vi "LINC Write Command (Raw).vi"(4 "raw byte offset (default)":i32=-1, 6 "timeout (2000)":u32=2000, 7 "parse only (F)":bool, 8 "error in (no error)":errorcluster, 9 "raw data":string, 10 "packet name":string, 11 "LINC session":refnum<class "LINC.lvclass">) -> (0 "error out":errorcluster, 1 "remote error":bool, 2 "binary command":string, 3 "dup LINC session":refnum<class "LINC.lvclass">)   [LabVIEW 2018, in "STEPkgDriver_LINC.lvlib" / "LINC.lvclass"]
uses:
  LINC.lvclass
  STEPkgDriver_LINC.lvlib
  LINC Global Session Mode.ctl
  LINC Global Config Mode.ctl
  LINC Global Handshake Mode.ctl
  LINC Handshake Internal.ctl
  LINC Global Mode.ctl
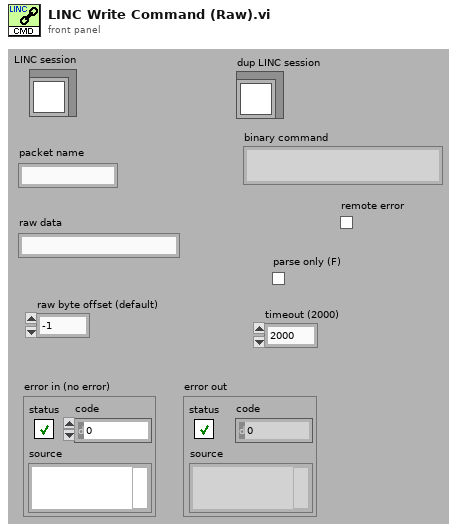
[diagram p1: front panel]
types:
  T1 = typedef "STEPkgDriver_LINC.lvlib/LINC Global Mode.ctl" = enum16{"INIT", "CLEAR", "ADD_PKT_HDR", "ADD_PKT", "GET_PKT_NAMES", "GET_PKT_DESC", "GET_PKT_HDR", "GET_PKT", "SET_PKT", "SET_DATA", "SIM_EN", "SIM_DS"}
  T2 = typedef "STEPkgDriver_LINC.lvlib/LINC Global Config Mode.ctl" = enum16{"INIT", "CLEAR", "SET_CMD_CB", "SET_TLM_CB", "SET_CMD_FIELDS", "SET_TLM_FIELDS", "SET_ID", "GET_CONFIG"}
  T3 = typedef "STEPkgDriver_LINC.lvlib/LINC Handshake Internal.ctl" = cluster{"error":errorcluster, "command data":string}
  T4 = typedef "STEPkgDriver_LINC.lvlib/LINC Global Handshake Mode.ctl" = enum16{"INIT", "CLEAR", "ADD_COMMAND", "RMV_COMMAND", "CLR_HANDSHAKE", "SET_HANDSHAKE", "GET_HANDSHAKE"}
  T5 = typedef "STEPkgDriver_LINC.lvlib/LINC Global Session Mode.ctl" = enum16{"INIT", "CLEAR", "ADD_SESSION", "SET_CONNECTION", "SET_LISTENER", "SET_REFERENCE", "GET_SESSION"}
  T6 = typedef "STEPkgDriver_LINC.lvlib/LINC Config.ctl" = cluster{"cmd callback":refnum<vi>, "tlm callback":refnum<vi>, "cmd ID bitoffset":i32, "cmd ID bitsize":i32, "cmd IDs":i32[], "tlm ID bitoffset":i32, "tlm ID bitsize":i32, "tlm IDs":i32[], "cmd header fields":i32, "tlm header fields":i32, "tlm header size":i32}
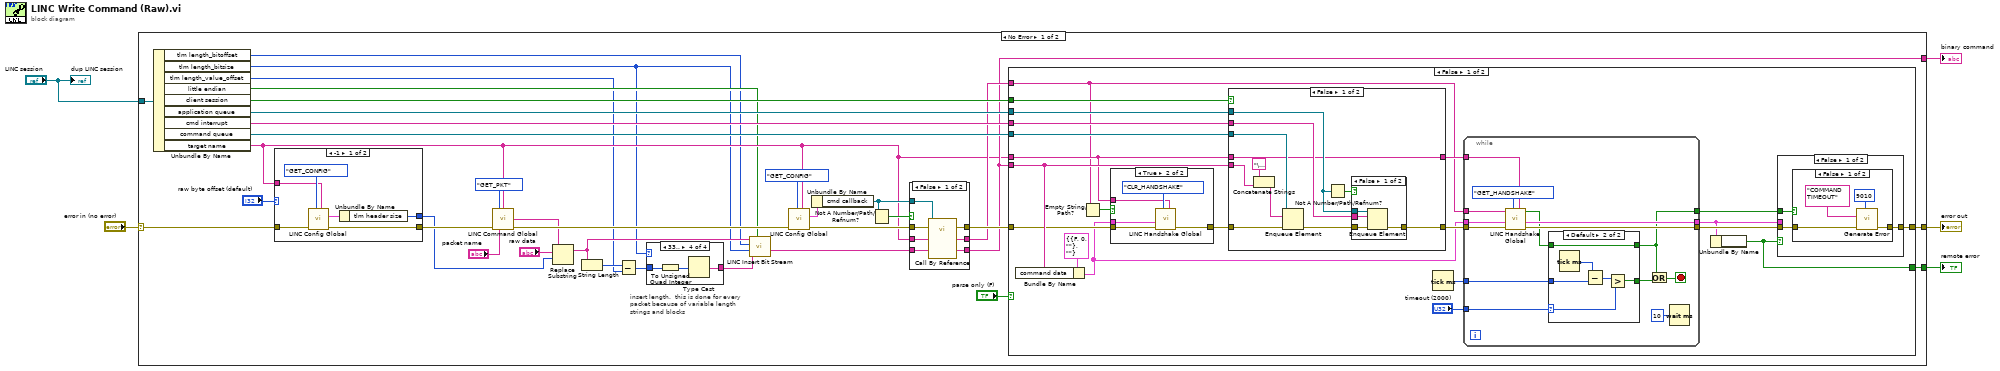
[diagram p0: block diagram]
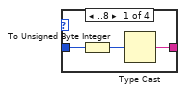
[diagram p2: hidden frame]
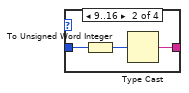
[diagram p3: hidden frame]
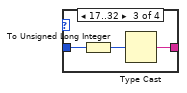
[diagram p4: hidden frame]
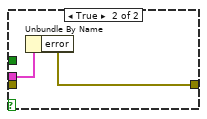
[diagram p8: hidden frame]
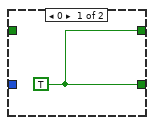
[diagram p10: hidden frame]
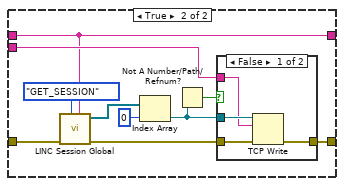
[diagram p12: hidden frame]
diagram:
  n1 = case shown="No Error" "error in (no error)" {
    selector: "error in (no error)" -> [w6 w160]
    tunnel: [w40 w160] -> w5
    tunnel: "LINC session" -> [w38 _]
    tunnel: [w26 _] -> w3
    tunnel: [w7 _] -> w2
    frame No Error {
      # "insert length.  this is done for every packet because of variable length strings and blocks"
      n2 = Unbundle By Name(w38) -> ("tlm length_bitoffset"=w8:i32, "tlm length_bitsize"=w9:i32, "tlm length_value_offset"=w10:i32, "little endian"=w11:bool, "client session"=w37:bool, "application queue"=w36:refnum<queue>, "cmd interrupt"=w35:string, "command queue"=w34:refnum<queue>, "target name"=w17:string)
      n3 = case shown="-1" "raw byte offset (default)" {
        selector: "raw byte offset (default)" -> [_ w59]
        tunnel: [w56 w60] -> w22
        tunnel: w6 -> [w55 w60]
        tunnel: [w54 w59] -> w18
        tunnel: w17 -> [w53 _]
        frame -1 {
          n4 = call "LINC Config Global.vi"("target name"=w53, "mode"=LINC_Global_Config_Mode."GET_CONFIG", "error in (no error)"=w55) -> ("error out"=w56:errorcluster, "config out"=w58:T6)  [unwired: 7 in]
          n5 = Unbundle By Name(w58) -> ("tlm header size"=w54:i32)
        }
        frame Default {
        }
      }
      n6 = call "LINC Command Global.vi"("mode"=LINC_Global_Mode."GET_PKT", "target name"=w17, "error in (no error)"=w22, "packet name"="packet name") -> ("data out"=w20:string, "error out"=w24:errorcluster)  [unwired: 7 in, 3 out]
      n7 = Replace Substring(3:w18, 4:"raw data", 5:w20) -> (1:w13:string)  [unwired: 1 in, 1 out]
      n8 = String Length(string=w13) -> (length=w14:i32)
      n9 = Subtract(x=w14, y=w10) -> (x-y=w15:i32)
      n10 = case shown="33.." w9 {
        tunnel: w15 -> [w42 w45 w48 w51]
        tunnel: [w41 w44 w47 w50] -> w16
        frame ..8 {
          n11 = To Unsigned Byte Integer(number=w42) -> (unsigned 8bit integer=w43:u8)
          n12 = Type Cast(x=w43) -> (*(type *) &x=w41:string)  [unwired: 1 in]
        }
        frame 9..16 {
          n13 = To Unsigned Word Integer(number=w45) -> (unsigned 16bit integer=w46:u16)
          n14 = Type Cast(x=w46) -> (*(type *) &x=w44:string)  [unwired: 1 in]
        }
        frame 17..32 {
          n15 = To Unsigned Long Integer(number=w48) -> (unsigned 32bit integer=w49:u32)
          n16 = Type Cast(x=w49) -> (*(type *) &x=w47:string)  [unwired: 1 in]
        }
        frame 33.. {
          n17 = To Unsigned Quad Integer(1:w51) -> (0:w52:u64)
          n18 = Type Cast(x=w52) -> (*(type *) &x=w50:string)  [unwired: 1 in]
        }
      }
      n19 = call "LINC Insert Bit Stream.vi"("little endian"=w11, "data to insert"=w16, "bit size"=w9, "bit offset"=w8, "data in"=w13) -> ("data out"=w12:string)  [unwired: 4 in]
      n20 = call "LINC Config Global.vi"("target name"=w17, "mode"=LINC_Global_Config_Mode."GET_CONFIG", "error in (no error)"=w24) -> ("error out"=w30:errorcluster, "config out"=w29:T6)  [unwired: 7 in]
      n21 = Unbundle By Name(w29) -> ("cmd callback"=w32:refnum<vi>)
      n22 = Not A Number/Path/Refnum?(number/path/refnum=w32) -> (NaN/Path/Refnum?=w31:bool)
      n23 = case shown="False" w31 {
        tunnel: [w67 w69] -> w28
        tunnel: w12 -> [w66 w68]
        tunnel: [w65 w68] -> w26
        tunnel: w30 -> [w64 w69]
        tunnel: w32 -> [w63 _]
        tunnel: w17 -> [w62 _]
        tunnel: [w61 _] -> w27
        frame False {
          n24 = call-by-ref "?"(reference=w63, error in=w64, "command in"=w66, "target name"=w62) -> (error out=w67:errorcluster, "command out"=w65:string, "GUID"=w61:string)  [unwired: 1 out]
        }
        frame True {
        }
      }
      n25 = case shown="False" "parse only (F)" {
        tunnel: [w72 w159] -> w40
        tunnel: w34 -> [w90 _]
        tunnel: w28 -> [w80 w159]
        tunnel: w26 -> [w81 _]
        tunnel: w35 -> [w89 _]
        tunnel: w36 -> [w88 _]
        tunnel: w37 -> [w87 _]
        tunnel: w17 -> [w78 _]
        tunnel: w27 -> [w76 _]
        tunnel: [w70 _] -> w7
        frame False {
          n26 = Bundle By Name(cluster=T3 {"error"={"status"=FALSE, "code"=0, "source"=""}, "command data"=""} ("handshake in"), "command data"=w81) -> (w77:T3)
          n27 = Empty String/Path?(string/path=w76) -> (empty?=w75:bool)
          n28 = case shown="True" w75 {
            tunnel: w80 -> [w101 w105]
            tunnel: [w101 w104] -> w79
            tunnel: w78 -> [_ w103]
            tunnel: w77 -> [_ w102]
            frame False {
            }
            frame True {
              n29 = call "LINC Handshake Global.vi"("target name"=w103, "mode"=LINC_Global_Handshake_Mode."CLR_HANDSHAKE", "error in (no error)"=w105, "handshake in"=w102) -> ("error out"=w104:errorcluster)  [unwired: 4 in, 3 out]
            }
          }
          n30 = case shown="False" w87 {
            tunnel: w90 -> [w138 _]
            tunnel: w79 -> [w136 w144]
            tunnel: w81 -> [w135 w150]
            tunnel: [w131 w153] -> w86
            tunnel: w89 -> [w130 _]
            tunnel: w88 -> [w129 _]
            tunnel: w78 -> [w128 w145]
            tunnel: [w128 w145] -> w85
            frame False {
              n31 = Concatenate Strings("\u0001" ("string"), w135) -> (w137:string)
              n32 = Enqueue Element(queue=w138, element=w137, error in (no error)=w136) -> (error out=w132:errorcluster)  [unwired: 1 in, 2 out]
              n33 = Not A Number/Path/Refnum?(number/path/refnum=w129) -> (NaN/Path/Refnum?=w133:bool)
              n34 = case shown="False" w133 {
                tunnel: w132 -> [w142 w143]
                tunnel: [w141 w143] -> w131
                tunnel: w129 -> [w140 _]
                tunnel: w130 -> [w139 _]
                frame False {
                  n35 = Enqueue Element(queue=w140, element=w139, error in (no error)=w142) -> (error out=w141:errorcluster)  [unwired: 1 in, 2 out]
                }
                frame True {
                }
              }
            }
            frame True {
              n36 = call "LINC Session Global.vi"("target name"=w145, "mode"=LINC_Global_Session_Mode."GET_SESSION", "error in (no error)"=w144) -> ("error out"=w152:errorcluster, "connections out"=w148:refnum<k5>[])  [unwired: 4 in, 3 out]
              n37 = Index Array(array=w148, index=0) -> (element=w146:refnum<k5>)
              n38 = Not A Number/Path/Refnum?(number/path/refnum=w146) -> (NaN/Path/Refnum?=w151:bool)
              n39 = case shown="False" w151 {
                tunnel: [w157 w158] -> w153
                tunnel: w152 -> [w156 w158]
                tunnel: w146 -> [w155 _]
                tunnel: w150 -> [w154 _]
                frame False {
                  n40 = TCP Write(connection ID=w155, data in=w154, error in (no error)=w156) -> (error out=w157:errorcluster)  [unwired: 1 in, 2 out]
                }
                frame True {
                }
              }
            }
          }
          n41 = Tick Count (ms)() -> (millisecond timer value=w84:u32)
          n42 = while {
            tunnel: w86 -> [w119]
            tunnel: [w118] -> w74
            tunnel: w85 -> [w117]
            tunnel: w76 -> [w116]
            tunnel: w84 -> [w115]
            tunnel: "timeout (2000)" -> [w112]
            tunnel: [w107] -> w71
            tunnel: w77 -> [w110]
            tunnel: [w109] -> w73
            stop <- w113 stop-if-true
            n43 = call "LINC Handshake Global.vi"("target name"=w117, "mode"=LINC_Global_Handshake_Mode."GET_HANDSHAKE", "error in (no error)"=w119, "handshake in"=w110, "GUID"=w116) -> ("error out"=w118:errorcluster, "handshake out"=w109:T3, "handshake"=w108:bool)  [unwired: 3 in, 1 out]
            n44 = case shown="Default" w112 {
              selector: w112 -> [_ w123]
              tunnel: w115 -> [_ w127]
              tunnel: [w121 w124] -> w111
              tunnel: w108 -> [_ w122]
              tunnel: [w121 w122] -> w107
              frame 0 {
                w121 = TRUE
              }
              frame Default {
                n45 = Tick Count (ms)() -> (millisecond timer value=w126:u32)
                n46 = Subtract(x=w126, y=w127) -> (x-y=w125:u32)
                n47 = Greater?(x=w125, y=w123) -> (0:w124:bool)
              }
            }
            n48 = Or(x=w107, y=w111) -> (x .or. y?=w113:bool)
            n49 = Wait (ms)(milliseconds to wait=u32 10) -> ()  [unwired: 1 out]
          }
          n50 = Unbundle By Name(w73) -> ("error.status"=w70:bool)
          n51 = case shown="False" w70 {
            tunnel: w74 -> [w93 _]
            tunnel: w73 -> [_ w100]
            tunnel: [w91 w99] -> w72
            tunnel: w71 -> [w92 _]
            frame False {
              n52 = case shown="False" w92 {
                tunnel: w93 -> [w97 w98]
                tunnel: [w96 w98] -> w91
                frame False {
                  n53 = call "Generate Error.vi"("error code (-1301)"=9010, "error in"=w97, "description"="COMMAND TIMEOUT") -> ("error out"=w96:errorcluster)  [unwired: 8 in]
                }
                frame True {
                }
              }
            }
            frame True {
              n54 = Unbundle By Name(w100) -> ("error"=w99:errorcluster)
            }
          }
        }
        frame True {
        }
      }
    }
    frame Error {
    }
  }
  "error out" <- w5
  "binary command" <- w3
  "remote error" <- w2
  "dup LINC session" <- "LINC session"
